vi "Num and Den from PFE.vi"(9 "Poles":cdb[](array[numeric]), 10 "Residues":cdb[][](array[numeric]), 11 "Multiplicity":i32[](array[numeric])) -> (0 "error":i32, 2 "Denominator":cdb[](array[numeric]), 3 "Numerator":cdb[](array[numeric]))   [LabVIEW 2014, in "NI_AALPro.lvlib"]
uses:
  NI_AALPro.lvlib
  Multiply Polynomials (CDB).vi
  Add Polynomials (CDB).vi
  Add Rational Polynomials (CDB).vi
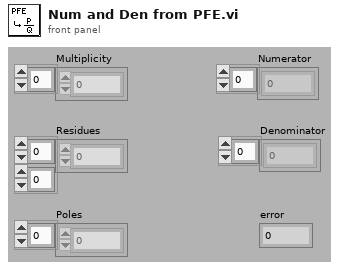
[diagram p1: front panel]
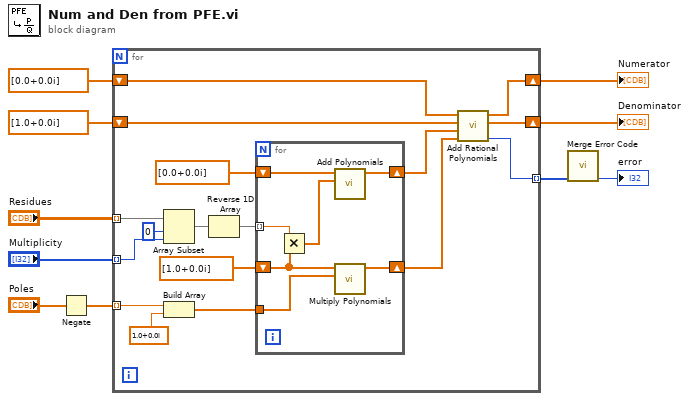
[diagram p0: block diagram]
diagram:
  n1 = Negate(x="Poles") -> (-x=w8:cdb[])
  n2 = for {
    tunnel: "Residues" -> [w22] mode=indexing
    shift-right: [w12] -> w5
    shift-left: cdb[] [0.0+0.0i] ("Numerator 1") -> [w26]
    shift-right: [w11] -> w6
    shift-left: cdb[] [1.0+0.0i] ("Numerator 1") -> [w25]
    tunnel: [w24] -> w1 mode=indexing
    tunnel: w8 -> [w23] mode=indexing
    tunnel: "Multiplicity" -> [w20] mode=indexing
    n3 = Array Subset(array=w22, index=0, length=w20) -> (w19:cdb[])
    n4 = Build Array(w23, cdb 1.0+0.0i ("element")) -> (w16:cdb[])
    n5 = Reverse 1D Array(array=w19) -> (reversed array=w18:cdb[])
    n6 = for {
      tunnel: w18 -> [w34] mode=indexing
      shift-right: [w31] -> w13
      shift-left: cdb[] [1.0+0.0i] ("Numerator 1") -> [w33]
      tunnel: w16 -> [w32]
      shift-right: [w28] -> w14
      shift-left: cdb[] [0.0+0.0i] ("Numerator 1") -> [w30]
      n7 = Multiply(x=w34, y=w33) -> (x*y=w29:cdb[])
      n8 = call-poly "Add Polynomials.vi"("Q(x)"=w29, "P(x)"=w30) -> ("P(x)+Q(x)"=w28:cdb[])  [unwired: 8 in, 1 out]
      n9 = call-poly "Multiply Polynomials.vi"("Q(x)"=w32, "P(x)"=w33) -> ("P(x)*Q(x)"=w31:cdb[])  [unwired: 8 in, 1 out]
    }
    n10 = call-poly "Add Rational Polynomials.vi"("Denominator 2"=w13, "Numerator 2"=w14, "Denominator 1"=w25, "Numerator 1"=w26) -> ("error"=w24:i32, "Denominator Out"=w11:cdb[], "Numerator Out"=w12:cdb[])  [unwired: 5 in]
  }
  "Denominator" <- w6
  "Numerator" <- w5
  n11 = call "Merge Error Code.vi"("Error Code"=w1) -> ("error code"=→"error":i32)  [unwired: 10 in]
